vi "list all modules.vi"(11 "resonant or galvo? (T is reso)":bool) -> (1 "inactive modules":string[](array[string]), 2 "optional modules":string[](array[string]), 3 "required modules":string[](array[string]))   [LabVIEW 2017]
doc: "SciScan 1.2 160622"
uses:
  GFG/GFGstringGet.vi
  GFG/GFG library.lvlib
panel:
  out "Numeric Control 2":i32
  out "Numeric Control":i32
  in  "error in (no error)":errorcluster
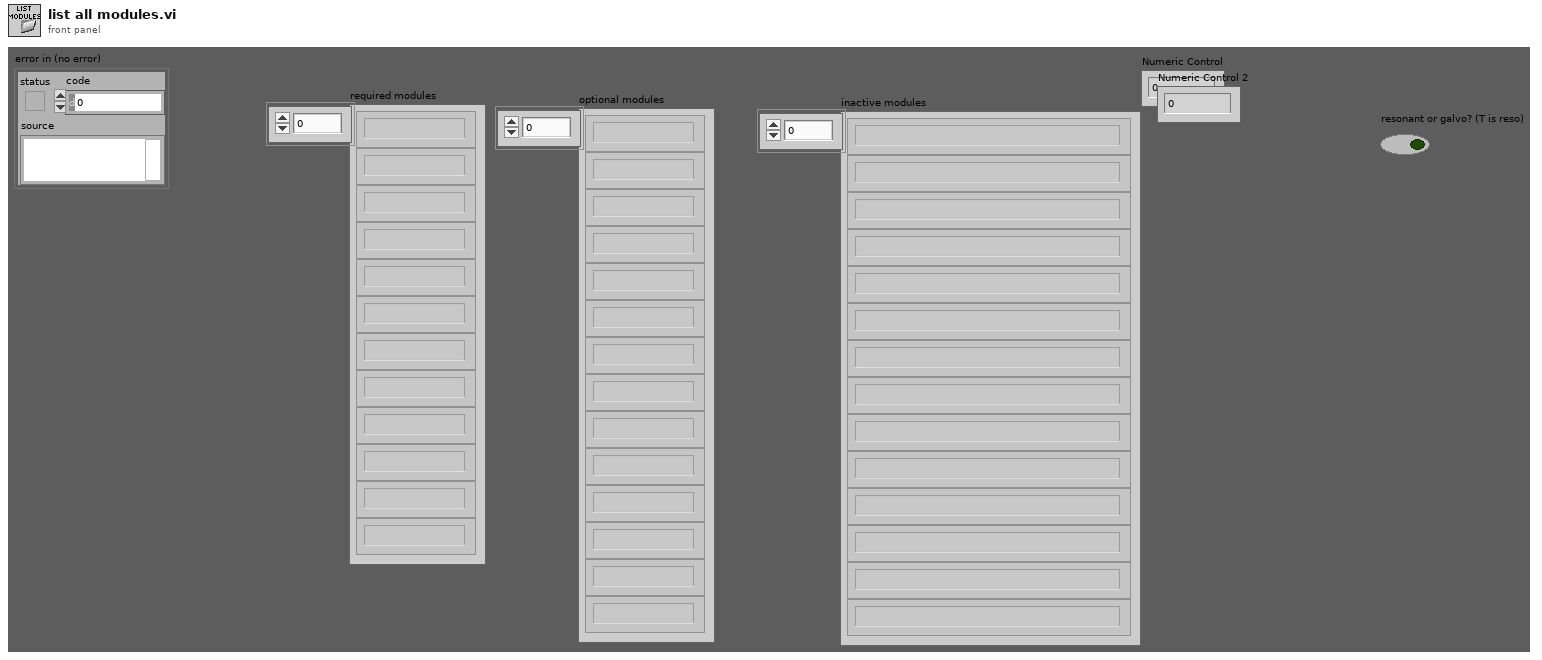
[diagram p1: front panel]
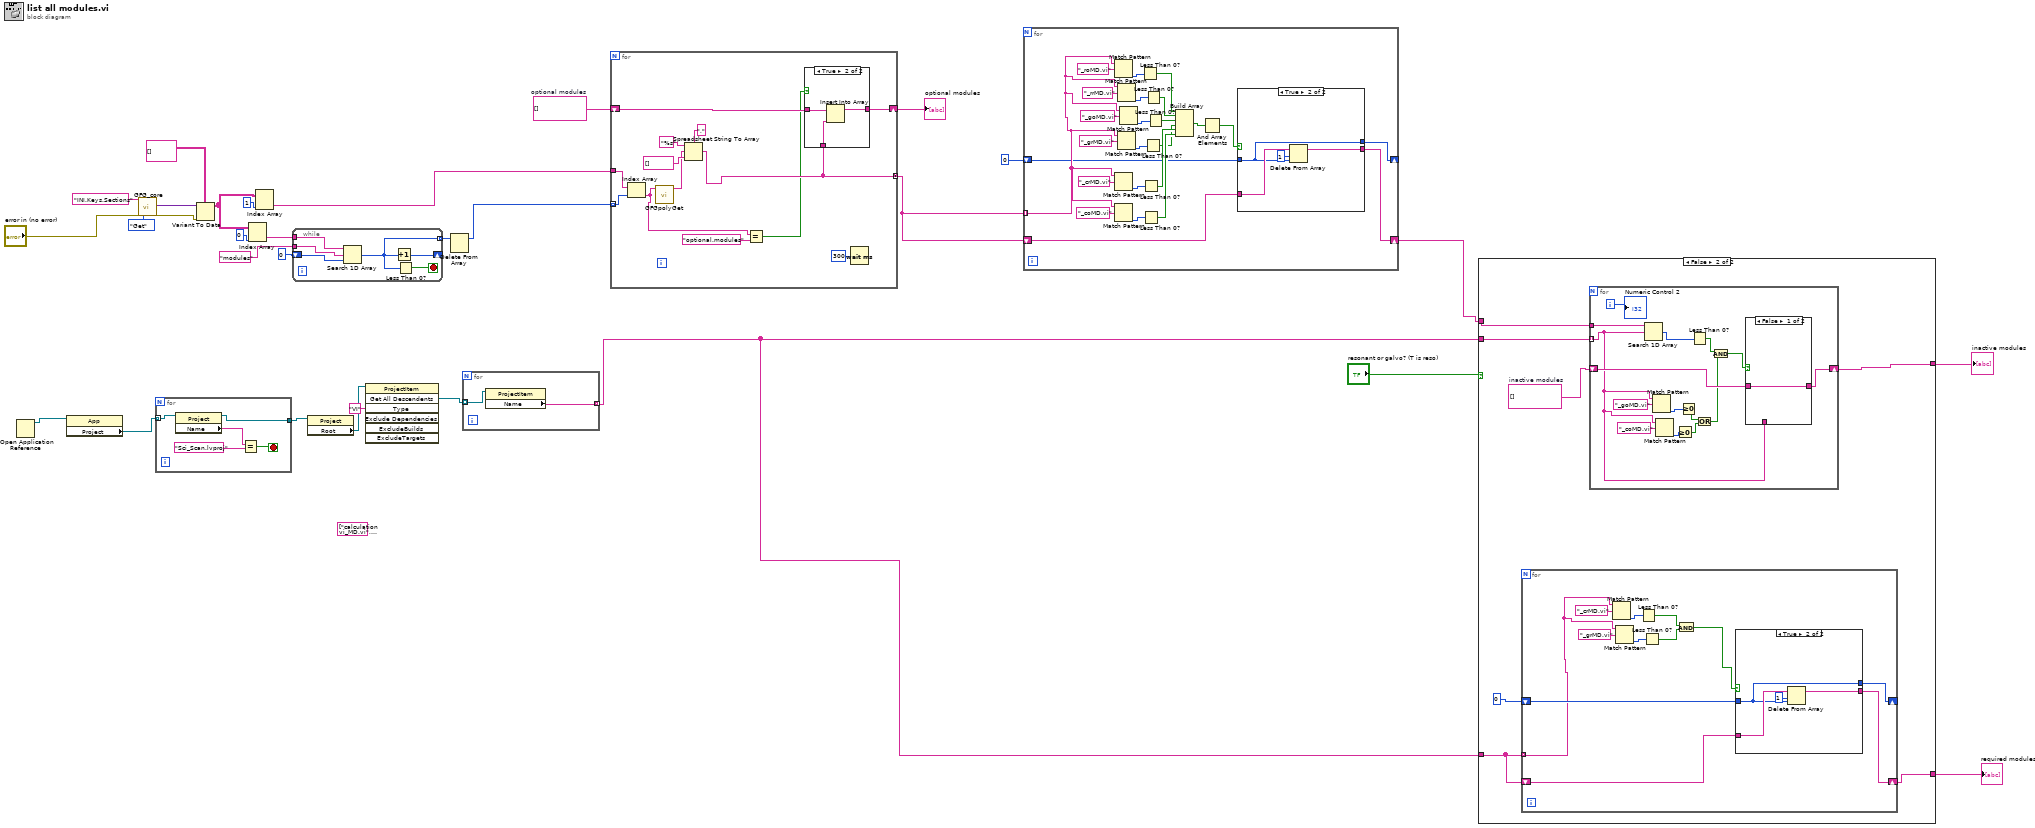
[diagram p0: block diagram]
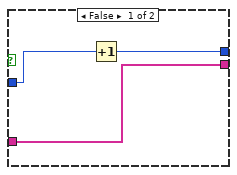
[diagram p2: hidden frame]
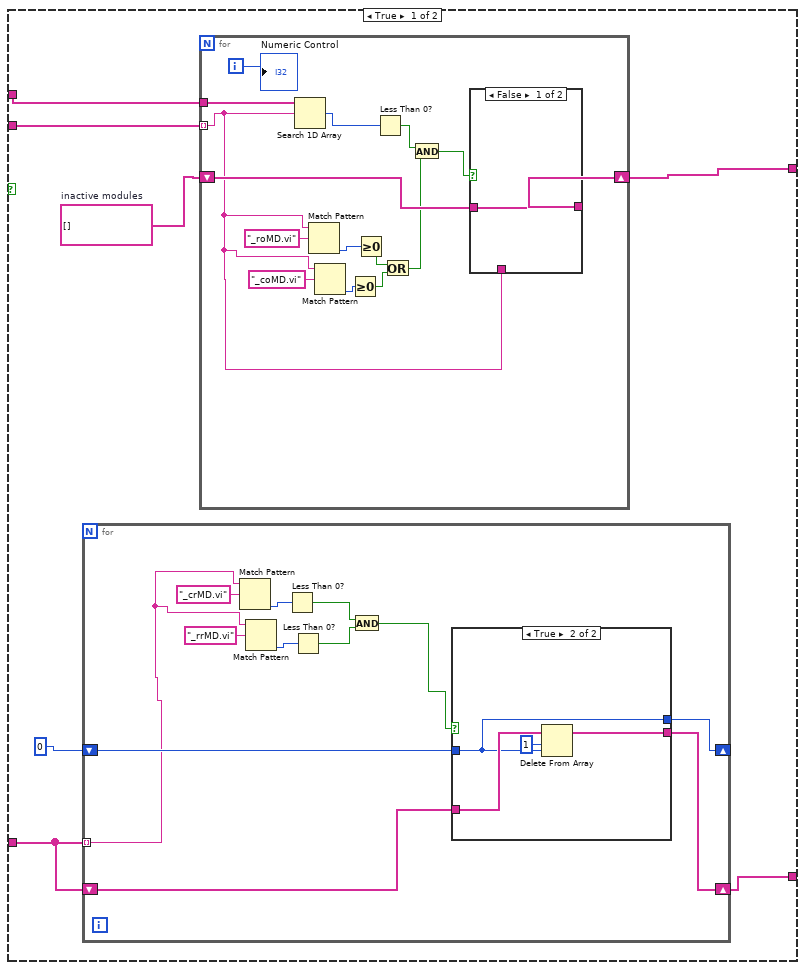
[diagram p3: hidden frame]
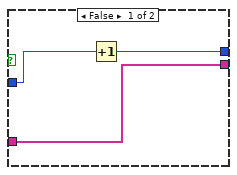
[diagram p4: hidden frame]
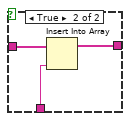
[diagram p5: hidden frame]
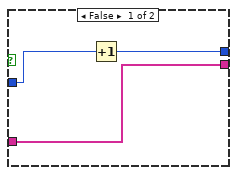
[diagram p6: hidden frame]
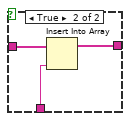
[diagram p7: hidden frame]
diagram:
  (unwired) string[] ["calculation vi_MD.vi", "XYZ stage handler_MD.vi", "galvo.scan.engine_MD.vi", "z.stack.run_MD.vi", "resonant.scan.engine_7962_MD.vi", "MIC communication_MD.vi", "MIC_MD.vi", "motorisedmirrors_MD.vi", "pockelscontrol_MD.vi", "pockelscontrol_w_blanking_for_PXI6259_MD.vi", "MOCK XYZ stage communication_MD.vi", "display queue to fp display_MD.vi", "image queue to disk and to display queue_MD.vi", "raw queue to image queue_MD.vi", "load_external_coordinates_MD.vi", "make arbitrary waveform_MD.vi", "standard frame scan geometry_MD.vi", "MacroLoopManager_MD.vi", "MacroOpsManager_MD.vi", "MacroStagePositioning_MD.vi", "Initialize_MacroGUI_MD.vi", "MacroGUI_MD.vi"] ("inactive modules")
  w13 = string[] []  # optional modules
  n1 = Open Application Reference() -> (3:w14:refnum<vi>)  [unwired: 4 in, 1 out]
  n2 = property class="App"(reference=w14) -> ("Project"=w15:refnum<vi>[])  [unwired: 1 in, 2 out]
  n3 = call "GFG_core.vi"("Variable Name in"="INI.Keys.Sections", "error in (no error)"="error in (no error)", "Action"=enum16{"Init", "Set", "Get"}."Get") -> ("Variant Out"=w28:variant, "error out"=w20:errorcluster)  [unwired: 10 in, 5 out]
  n4 = for {
    tunnel: w15 -> [w35] mode=indexing
    tunnel: [w32] -> w16
    stop <- w31 stop-if-true
    n5 = property class="Project"(reference=w35) -> (reference out=w32:refnum<vi>, "Name"=w33:string)  [unwired: 1 in, 1 out]
    n6 = Equal?(x=w33, y="Sci_Scan.lvproj" ("Name")) -> (x = y?=w31:bool)
  }
  n7 = Variant To Data(error in=w20, type=string[][] [], Variant=w28) -> (data=w11:string[][])  [unwired: 1 out]
  n8 = Index Array(array=w11, index (col)=0 ("index (row)")) -> (element=w19:string[])  [unwired: 1 in]
  n9 = Index Array(array=w11, index (col)=1 ("index (row)")) -> (element=w17:string[])  [unwired: 1 in]
  n10 = while {
    tunnel: w19 -> [w41]
    shift-right: [w38] -> _
    shift-left: 0 ("index of element") -> [w40]
    tunnel: [w37] -> w22 mode=indexing
    tunnel: "modules" ("element") -> [w36]
    stop <- w39 stop-if-true
    n11 = Search 1D Array(1D array=w41, element=w36, start index (0)=w40) -> (index of element=w37:i32)
    n12 = Increment(x=w37) -> (x+1=w38:i32)
    n13 = Less Than 0?(x=w37) -> (x < 0?=w39:bool)
  }
  n14 = property class="Project"(reference=w16) -> ("Root"=w10:refnum<vi>)  [unwired: 1 in, 2 out]
  n15 = invoke class="ProjectItem" method="Get All Descendents"(reference=w10, "Type"="VI") -> ("All Descendents"=w8:refnum<vi>[])  [unwired: 5 in, 6 out]
  n16 = Delete From Array(array=w22) -> (array with subset deleted=w18:i32[])  [unwired: 2 in, 1 out]
  n17 = for {
    tunnel: w8 -> [w43] mode=indexing
    tunnel: [w42] -> w2 mode=indexing
    n18 = property class="ProjectItem"(reference=w43) -> ("Name"=w42:string)  [unwired: 1 in, 2 out]
  }
  n19 = for {
    tunnel: w17 -> [w56]
    tunnel: w18 -> [w51] mode=indexing
    tunnel: [w48] -> w5 mode=concatenating
    shift-right: [w47] -> w12
    shift-left: w13 -> [w49]
    n20 = Index Array(array=w56, index=w51) -> (element=w45:string)
    n21 = call-poly "GFGpolyGet.vi"("Variable Name in"=w45) -> ("String"=w52:string)  [unwired: 9 in, 1 out]
    n22 = Spreadsheet String To Array(delimiter (Tab)=",", format string="%s" ("Variable Name in"), spreadsheet string=w52, array type (2D Dbl)=string[] [] ("Array")) -> (array=w48:string[])
    n23 = Equal?(x=w45, y="optional.modules") -> (x = y?=w46:bool)
    n24 = case shown="True" w46 {
      tunnel: w49 -> [w57 w60]
      tunnel: w48 -> [_ w59]
      tunnel: [w57 w58] -> w47
      frame False {
      }
      frame True {
        n25 = Insert Into Array(array=w60, new element=w59) -> (w58:string[])  [unwired: 1 in]
      }
    }
    n26 = Wait (ms)(milliseconds to wait=u32 300) -> ()  [unwired: 1 out]
  }
  "optional modules" <- w12
  n27 = for {
    tunnel: w5 -> [w66] mode=indexing
    shift-right: [w62] -> _
    shift-left: 0 -> [w63]
    shift-right: [w61] -> w3
    shift-left: w5 -> [w64]
    n28 = Match Pattern(string=w66, regular expression="_roMD.vi") -> (offset past match=w68:i32)  [unwired: 1 in, 3 out]
    n29 = Match Pattern(string=w66, regular expression="_crMD.vi") -> (offset past match=w76:i32)  [unwired: 1 in, 3 out]
    n30 = Match Pattern(string=w66, regular expression="_coMD.vi") -> (offset past match=w77:i32)  [unwired: 1 in, 3 out]
    n31 = Match Pattern(string=w66, regular expression="_grMD.vi") -> (offset past match=w73:i32)  [unwired: 1 in, 3 out]
    n32 = Match Pattern(string=w66, regular expression="_rrMD.vi") -> (offset past match=w69:i32)  [unwired: 1 in, 3 out]
    n33 = Match Pattern(string=w66, regular expression="_goMD.vi") -> (offset past match=w72:i32)  [unwired: 1 in, 3 out]
    n34 = Less Than 0?(x=w68) -> (x < 0?=w85:bool)
    n35 = Less Than 0?(x=w76) -> (x < 0?=w82:bool)
    n36 = Less Than 0?(x=w77) -> (x < 0?=w83:bool)
    n37 = Less Than 0?(x=w73) -> (x < 0?=w81:bool)
    n38 = Less Than 0?(x=w69) -> (x < 0?=w79:bool)
    n39 = Less Than 0?(x=w72) -> (x < 0?=w80:bool)
    n40 = Build Array(w85, w79, w80, w81, w82, w83) -> (w84:bool[])
    n41 = And Array Elements(Boolean array=w84) -> (logical AND=w65:bool)
    n42 = case shown="True" w65 {
      tunnel: w64 -> [w86 w92]
      tunnel: w63 -> [w88 w90]
      tunnel: [w87 w90] -> w62
      tunnel: [w86 w89] -> w61
      frame False {
        n43 = Increment(x=w88) -> (x+1=w87:i32)
      }
      frame True {
        n44 = Delete From Array(array=w92, length=1, index=w90) -> (array with subset deleted=w89:string[])  [unwired: 1 out]
      }
    }
  }
  n45 = case shown="False" "resonant or galvo? (T is reso)" {
    tunnel: w3 -> [w99 w144]
    tunnel: w2 -> [w97 w142]
    tunnel: [w96 w141] -> w6
    tunnel: w2 -> [w94 w139]
    tunnel: [w93 w138] -> w1
    frame True {
      w98 = string[] []  # inactive modules
      n46 = for {
        tunnel: w94 -> [w103] mode=indexing
        shift-right: [w105] -> _
        shift-left: 0 -> [w106]
        shift-right: [w104] -> w93
        shift-left: w94 -> [w107]
        n47 = Match Pattern(string=w103, regular expression="_crMD.vi") -> (offset past match=w109:i32)  [unwired: 1 in, 3 out]
        n48 = Match Pattern(string=w103, regular expression="_rrMD.vi") -> (offset past match=w110:i32)  [unwired: 1 in, 3 out]
        n49 = Less Than 0?(x=w109) -> (x < 0?=w102:bool)
        n50 = Less Than 0?(x=w110) -> (x < 0?=w101:bool)
        n51 = And(x=w102, y=w101) -> (x .and. y?=w100:bool)
        n52 = case shown="True" w100 {
          tunnel: w107 -> [w112 w118]
          tunnel: w106 -> [w114 w116]
          tunnel: [w113 w116] -> w105
          tunnel: [w112 w115] -> w104
          frame False {
            n53 = Increment(x=w114) -> (x+1=w113:i32)
          }
          frame True {
            n54 = Delete From Array(array=w118, length=1, index=w116) -> (array with subset deleted=w115:string[])  [unwired: 1 out]
          }
        }
      }
      n55 = for {
        tunnel: w97 -> [w125] mode=indexing
        tunnel: w99 -> [w133]
        shift-right: [w131] -> w96
        shift-left: w98 -> [w132]
        i -> [w128]
        n56 = Search 1D Array(1D array=w133, element=w125) -> (index of element=w124:i32)  [unwired: 1 in]
        n57 = Match Pattern(string=w125, regular expression="_roMD.vi") -> (offset past match=w129:i32)  [unwired: 1 in, 3 out]
        n58 = Match Pattern(string=w125, regular expression="_coMD.vi") -> (offset past match=w127:i32)  [unwired: 1 in, 3 out]
        n59 = Greater Or Equal To 0?(x=w127) -> (x >= 0?=w122:bool)
        n60 = Greater Or Equal To 0?(x=w129) -> (x >= 0?=w123:bool)
        n61 = Less Than 0?(x=w124) -> (x < 0?=w121:bool)
        n62 = Or(x=w123, y=w122) -> (x .or. y?=w120:bool)
        n63 = And(x=w121, y=w120) -> (x .and. y?=w119:bool)
        n64 = case shown="False" w119 {
          tunnel: w132 -> [w134 w137]
          tunnel: w125 -> [_ w136]
          tunnel: [w134 w135] -> w131
          frame False {
          }
          frame True {
            n65 = Insert Into Array(array=w137, new element=w136) -> (w135:string[])  [unwired: 1 in]
          }
        }
        "Numeric Control" <- w128
      }
    }
    frame False {
      w143 = string[] []  # inactive modules
      n66 = for {
        tunnel: w139 -> [w148] mode=indexing
        shift-right: [w150] -> _
        shift-left: 0 -> [w151]
        shift-right: [w149] -> w138
        shift-left: w139 -> [w152]
        n67 = Match Pattern(string=w148, regular expression="_crMD.vi") -> (offset past match=w154:i32)  [unwired: 1 in, 3 out]
        n68 = Match Pattern(string=w148, regular expression="_grMD.vi") -> (offset past match=w155:i32)  [unwired: 1 in, 3 out]
        n69 = Less Than 0?(x=w154) -> (x < 0?=w147:bool)
        n70 = Less Than 0?(x=w155) -> (x < 0?=w146:bool)
        n71 = And(x=w147, y=w146) -> (x .and. y?=w145:bool)
        n72 = case shown="True" w145 {
          tunnel: w152 -> [w157 w163]
          tunnel: w151 -> [w159 w161]
          tunnel: [w158 w161] -> w150
          tunnel: [w157 w160] -> w149
          frame False {
            n73 = Increment(x=w159) -> (x+1=w158:i32)
          }
          frame True {
            n74 = Delete From Array(array=w163, length=1, index=w161) -> (array with subset deleted=w160:string[])  [unwired: 1 out]
          }
        }
      }
      n75 = for {
        tunnel: w142 -> [w170] mode=indexing
        tunnel: w144 -> [w178]
        shift-right: [w176] -> w141
        shift-left: w143 -> [w177]
        i -> [w173]
        n76 = Search 1D Array(1D array=w178, element=w170) -> (index of element=w169:i32)  [unwired: 1 in]
        n77 = Match Pattern(string=w170, regular expression="_goMD.vi") -> (offset past match=w174:i32)  [unwired: 1 in, 3 out]
        n78 = Match Pattern(string=w170, regular expression="_coMD.vi") -> (offset past match=w172:i32)  [unwired: 1 in, 3 out]
        n79 = Greater Or Equal To 0?(x=w172) -> (x >= 0?=w167:bool)
        n80 = Greater Or Equal To 0?(x=w174) -> (x >= 0?=w168:bool)
        n81 = Less Than 0?(x=w169) -> (x < 0?=w166:bool)
        n82 = Or(x=w168, y=w167) -> (x .or. y?=w165:bool)
        n83 = And(x=w166, y=w165) -> (x .and. y?=w164:bool)
        n84 = case shown="False" w164 {
          tunnel: w177 -> [w179 w182]
          tunnel: w170 -> [_ w181]
          tunnel: [w179 w180] -> w176
          frame False {
          }
          frame True {
            n85 = Insert Into Array(array=w182, new element=w181) -> (w180:string[])  [unwired: 1 in]
          }
        }
        "Numeric Control 2" <- w173
      }
    }
  }
  "required modules" <- w1
  "inactive modules" <- w6
